vi "Set Numeric Text.vi"(7 "Treatment of Infinity/NaN":T1, 8 "error in (no error)":errorcluster, 10 "Numeric Text":string, 11 "JSON Scalar in":refnum<class "JSON Scalar.lvclass">) -> (0 "error out":errorcluster, 3 "JSON Scalar out":refnum<class "JSON Scalar.lvclass">)   [LabVIEW 2011, in "JSON Scalar.lvclass"]
uses:
  JSON Scalar.lvclass
  Infinity&NaN.ctl
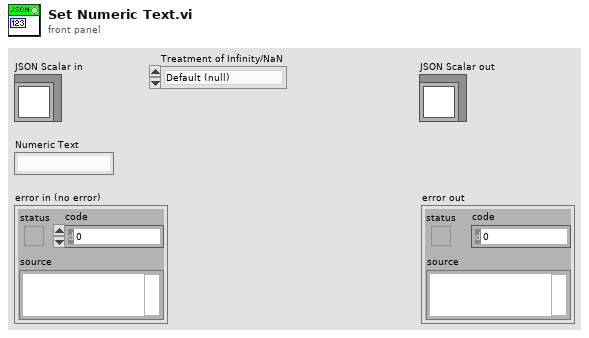
[diagram p1: front panel]
types:
  T1 = typedef "JSON Scalar.lvclass/Infinity&NaN.ctl" = enum16{"Default (null)", "Extended", "LabVIEW extensions"}
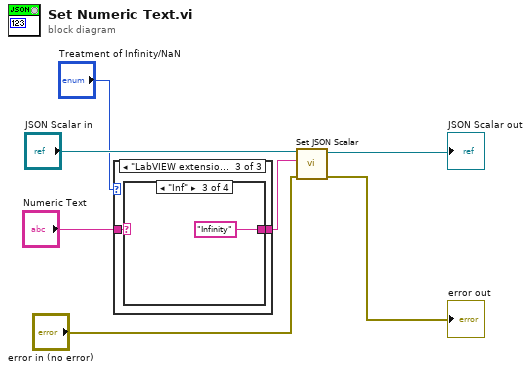
[diagram p0: block diagram]
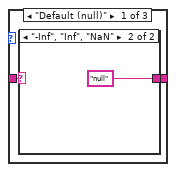
[diagram p2: hidden frame]
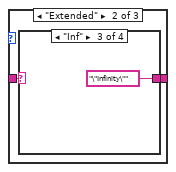
[diagram p4: hidden frame]
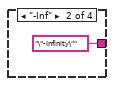
[diagram p6: hidden frame]
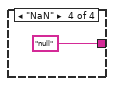
[diagram p7: hidden frame]
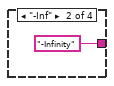
[diagram p9: hidden frame]
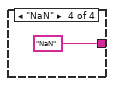
[diagram p10: hidden frame]
diagram:
  n1 = case shown="\"LabVIEW extensions\"" "Treatment of Infinity/NaN" {
    tunnel: "Numeric Text" -> [w9 w13 w19]
    tunnel: [w8 w12 w18] -> w2
    frame "Default (null)" {
      n2 = case shown="\"-Inf\", \"Inf\", \"NaN\"" w9 {
        selector: w9 -> [w10 _]
        tunnel: [w10 "null"] -> w8
        frame Default {
        }
        frame "-Inf", "Inf", "NaN" {
        }
      }
    }
    frame "Extended" {
      n3 = case shown="\"Inf\"" w13 {
        selector: w13 -> [w14 _ _ _]
        tunnel: [w14 "\"-Infinity\"" "\"Infinity\"" "null"] -> w12
        frame Default {
        }
        frame "-Inf" {
        }
        frame "Inf" {
        }
        frame "NaN" {
        }
      }
    }
    frame "LabVIEW extensions" {
      n4 = case shown="\"Inf\"" w19 {
        selector: w19 -> [w20 _ _ _]
        tunnel: [w20 "-Infinity" "Infinity" "NaN"] -> w18
        frame Default {
        }
        frame "-Inf" {
        }
        frame "Inf" {
        }
        frame "NaN" {
        }
      }
    }
  }
  n5 = call "Set JSON Scalar.vi"("error in (no error)"="error in (no error)", "LabVIEW Text"=w2, "JSON Scalar in"="JSON Scalar in") -> ("error out"=→"error out":errorcluster, "JSON Scalar out"=→"JSON Scalar out":refnum<class "JSON Scalar.lvclass">)  [unwired: 7 in]
